vi "Get Ramping Mode.vi"(0 "VISA resource name":refnum<visa-resource-name>, 1 "error in":T1) -> (2 "VISA resource name out":refnum<visa-resource-name>, 3 "Ramping Mode String":string, 4 "Ramping Mode":T2(ring)=enum."RAMPING", 5 "error out":T1)   [LabVIEW 2019]
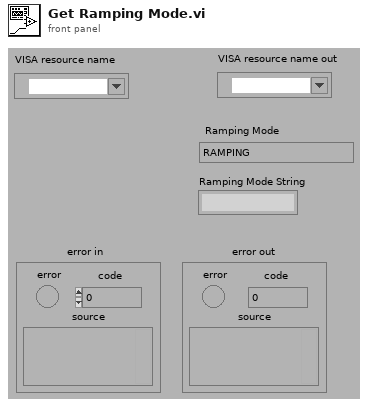
[diagram p1: front panel]
types:
  T1 = cluster{"error":bool, "code":i32, "source":string}
  T2 = enum16{"", "RAMPING", "HOLDING", "PAUSED", "MANUAL UP", "MANUAL DOWN", "ZEROING CURRENT", "QUENCH DETECTED", "AT ZERO", "HEATING SWITCH", "COOLING SWITCH", "EXTERNAL RAMPDOWN"}
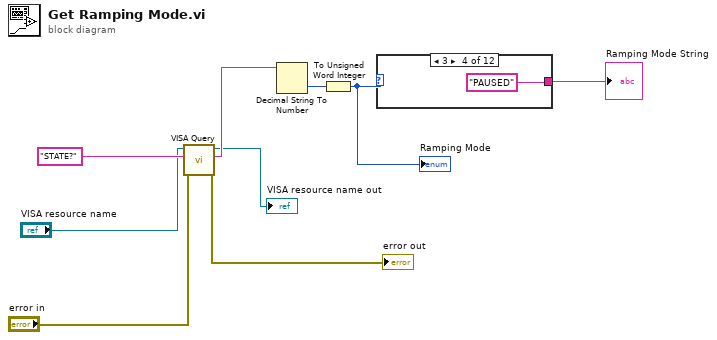
[diagram p0: block diagram]
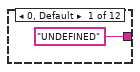
[diagram p2: hidden frame]
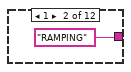
[diagram p3: hidden frame]
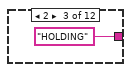
[diagram p4: hidden frame]
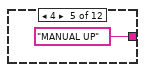
[diagram p5: hidden frame]
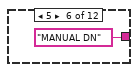
[diagram p6: hidden frame]
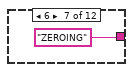
[diagram p7: hidden frame]
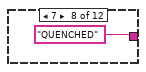
[diagram p8: hidden frame]
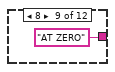
[diagram p9: hidden frame]
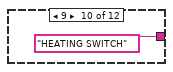
[diagram p10: hidden frame]
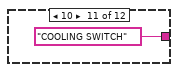
[diagram p11: hidden frame]
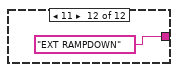
[diagram p12: hidden frame]
diagram:
  n1 = call "VISA Query.vi"("error in (no error)"="error in", "Command"="STATE?", "VISA resource name"="VISA resource name") -> ("error out"=→"error out":errorcluster, "Response"=w5:string, "VISA resource name out"=→"VISA resource name out":refnum<visa-resource-name>)  [unwired: 4 in, 2 out]
  n2 = Decimal String To Number(string=w5) -> (number=w4:i32)  [unwired: 2 in, 1 out]
  n3 = To Unsigned Word Integer(number=w4) -> (unsigned 16bit integer=w3:u16)
  "Ramping Mode" <- w3
  n4 = case shown="3" w3 {
    tunnel: ["UNDEFINED" ("string") "RAMPING" ("string") "HOLDING" ("string") "PAUSED" ("string") "MANUAL UP" ("string") "MANUAL DN" ("string") "ZEROING" ("string") "QUENCHED" ("string") "AT ZERO" ("string") "HEATING SWITCH" ("string") "COOLING SWITCH" ("string") "EXT RAMPDOWN" ("string")] -> w6
    frame 0, Default {
    }
    frame 1 {
    }
    frame 2 {
    }
    frame 3 {
    }
    frame 4 {
    }
    frame 5 {
    }
    frame 6 {
    }
    frame 7 {
    }
    frame 8 {
    }
    frame 9 {
    }
    frame 10 {
    }
    frame 11 {
    }
  }
  "Ramping Mode String" <- w6
